vi "G Code Commands.vi"(4 "Previous G Code":T1, 6 "Current G Code":T1, 8 "Error In":errorcluster, 9 "Fast Velocity(mm/s)":dbl=80.0, 10 "Coordinate Space Reference In":refnum<k21>, 11 "Axis Resources In":refnum<k21>[](array[refnum])=["", "", "", ""]) -> (0 "Error Out":errorcluster, 2 "Coordinate Space Reference Out":refnum<k21>, 3 "Axis Resources Out":refnum<k21>[](array[refnum]))   [LabVIEW 2018]
uses:
  Type Defs/G Code Command Cluster.ctl
  Type Defs/The Motion Parameters.ctl
  <vilib>/Motion/Express/_s/nimc.ex.straightLineMove.startStraightLineMove.coordinate.modeAbsolute.blendEnable.1.vi
  <vilib>/Motion/Express/_s/nimc.ex.arcMove.startArcMove.coordinate.modeCircular.blendEnable.1.vi
  <vilib>/Motion/Express/_s/nimc.ex.stopMove.stop.axis.modeDecelerate.vi
  <vilib>/Motion/Express/_s/nimc.ex.resetPosition.resetPosition.axis.vi
  <vilib>/Motion/BlockNode/FB.NIMotion.xnode
  <vilib>/Motion/Express/_s/nimc.fb.straightLineMove.blendMode.ctl
  <vilib>/Motion/Express/_s/nimc.fb.arcMove.blendMode.ctl
panel:
  in  "Dwell Time(ms)":u32
  in  "Motion Parameters":T2={"Timeout"=-1.0, "Blend Mode"=10551335, "Acceleration"=2000.0, "Deceleration"=2000.0, "Accel. Jerk"=20000.0, "Decel. Jerk"=20000.0, "Smoothing"=1.0, "Last Blend"=FALSE, "Blend Delay"=0.0} {"Blend Delay" format="%#_13g"; "Smoothing" format="%#_13g"; "Decel. Jerk" format="%#_13g"; "Accel. Jerk" format="%#_13g"; "Deceleration" format="%#_13g"; "Acceleration" format="%#_13g"; "Blend Mode" items=["At Profile Complete"=10551335, "At Deceleration"=10551334, "After Delay"=10551336]}
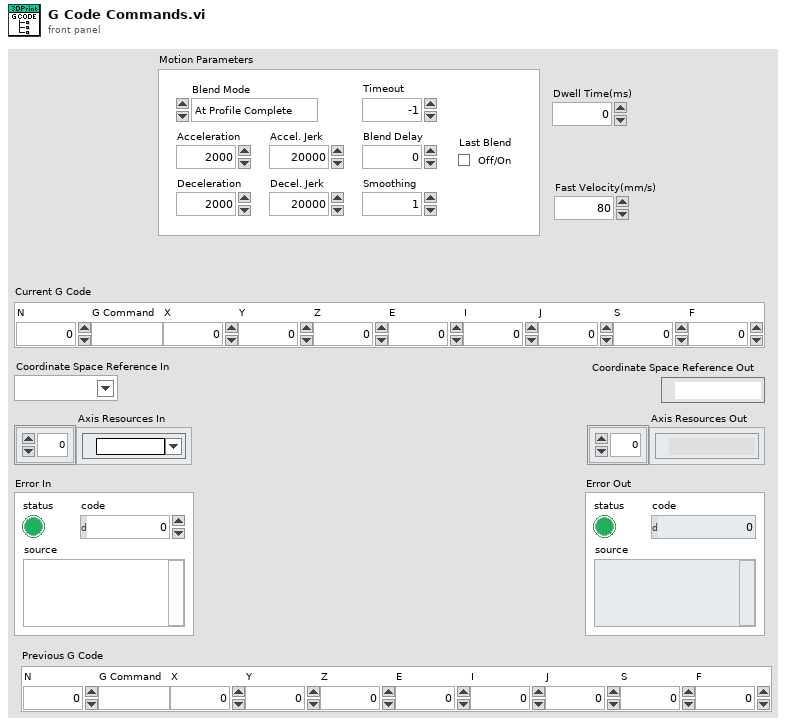
[diagram p1: front panel]
types:
  T1 = typedef "G Code Command Cluster.ctl" = cluster{"N":dbl, "G Command":string, "X":dbl, "Y":dbl, "Z":dbl, "E":dbl, "I":dbl, "J":dbl, "S":dbl, "F":dbl}
  T2 = typedef "The Motion Parameters.ctl" = cluster{"Timeout":dbl, "Blend Mode":i32, "Acceleration":dbl, "Deceleration":dbl, "Accel. Jerk":dbl, "Decel. Jerk":dbl, "Smoothing":dbl, "Last Blend":bool, "Blend Delay":dbl}
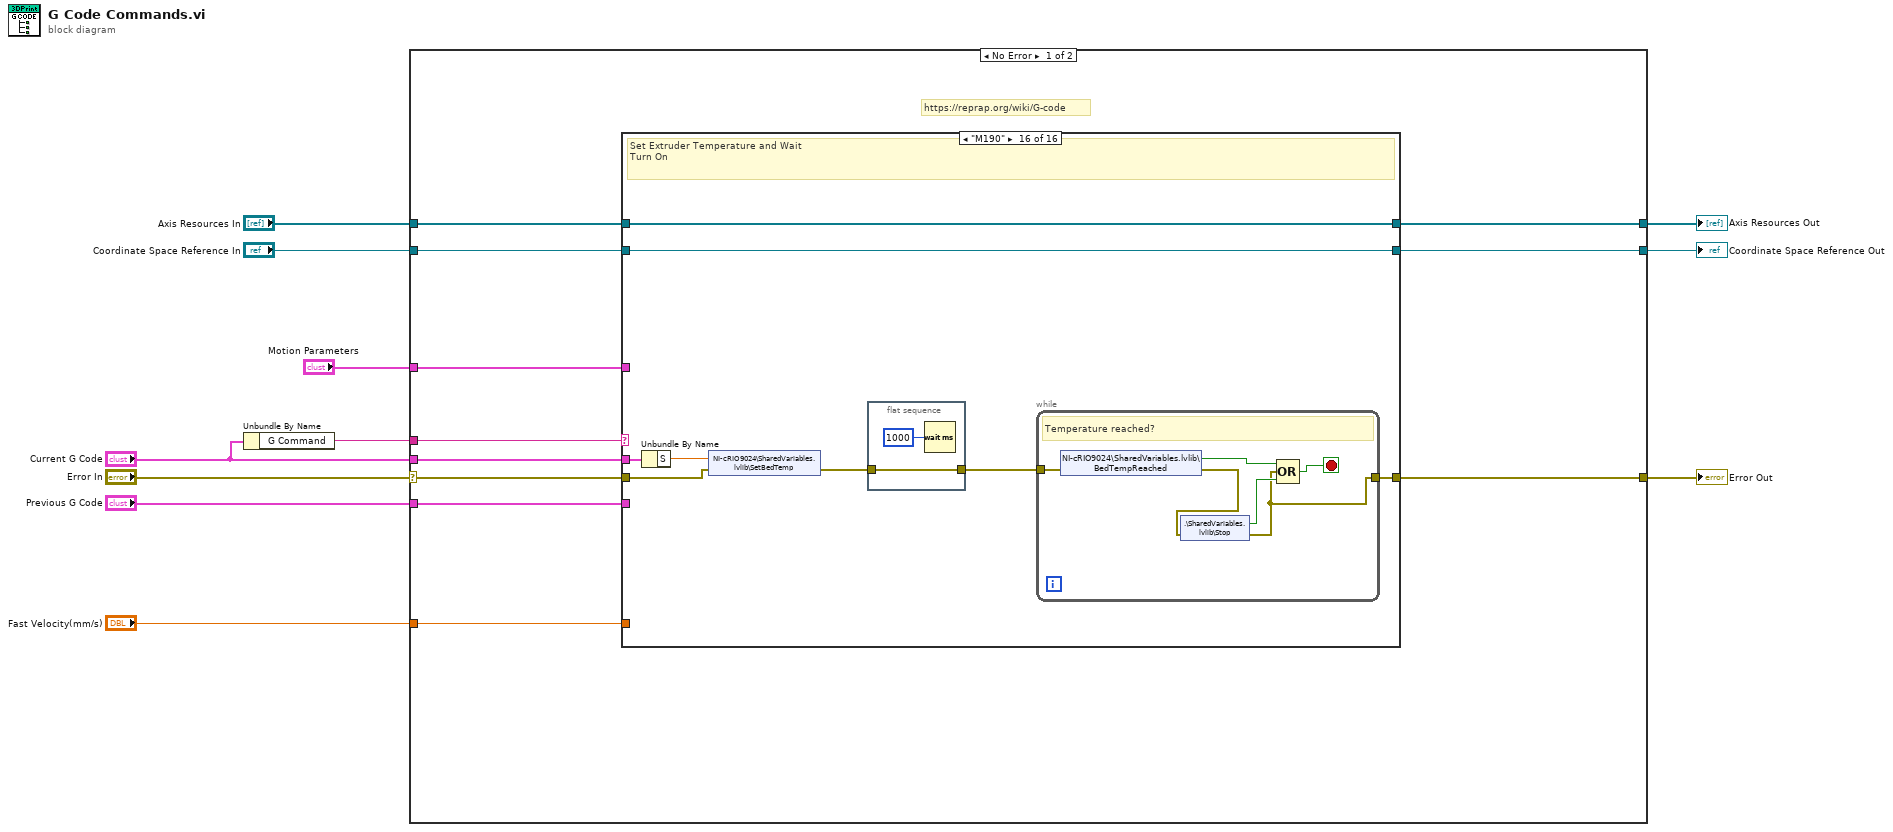
[diagram p0: block diagram]
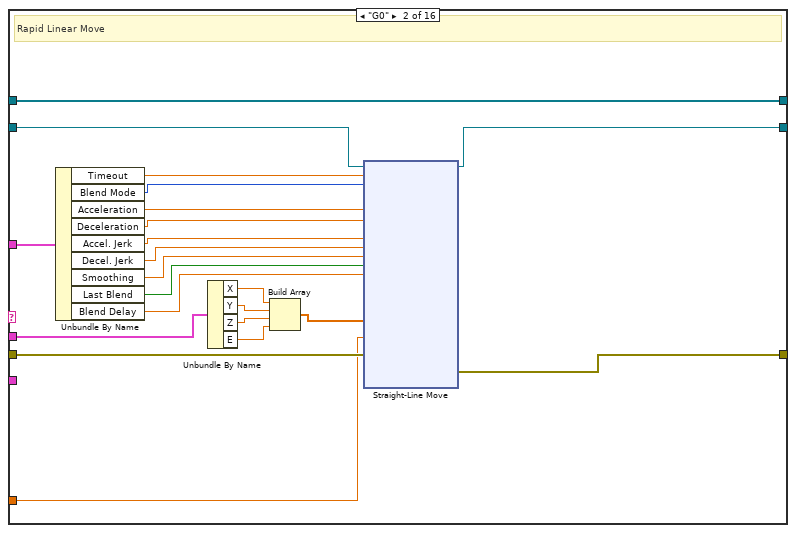
[diagram p3: hidden frame]
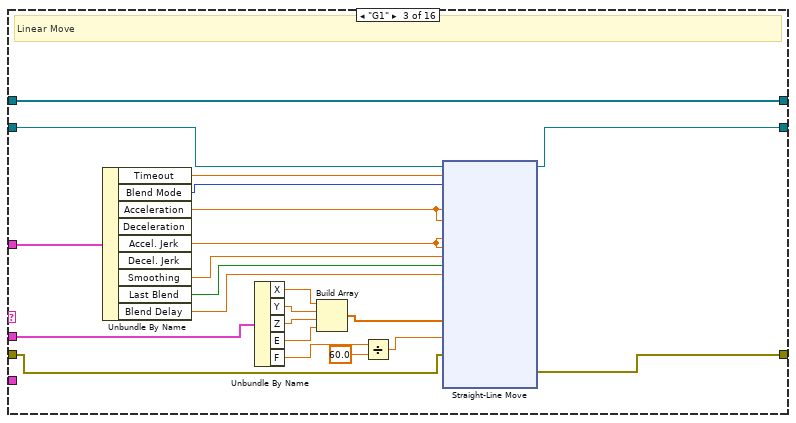
[diagram p4: hidden frame]
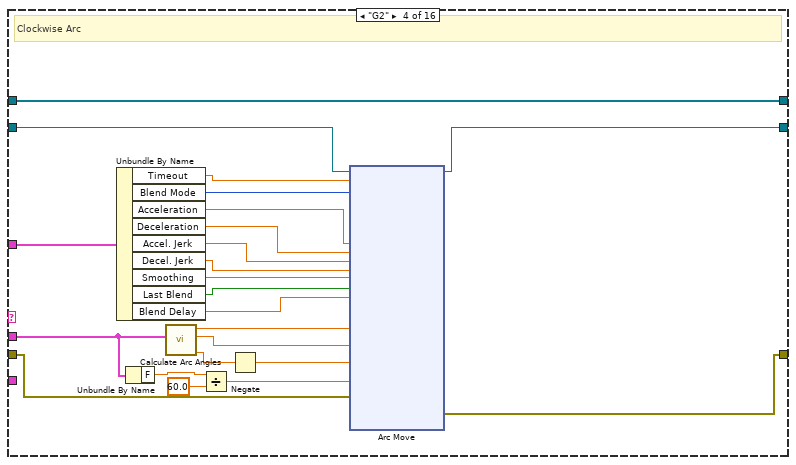
[diagram p5: hidden frame]
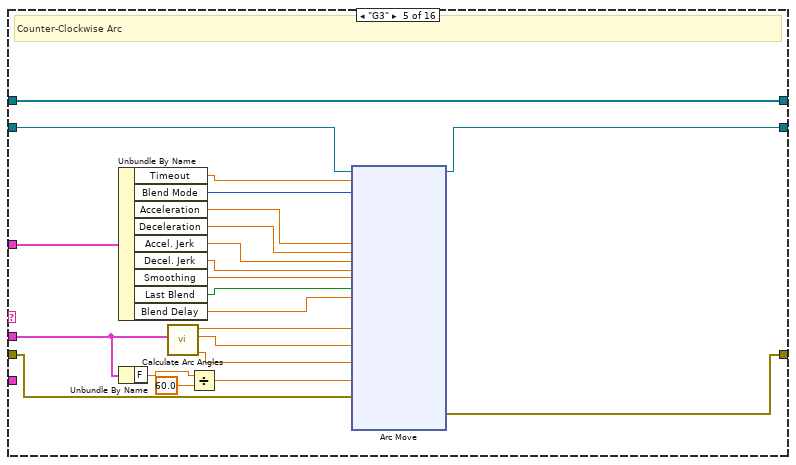
[diagram p6: hidden frame]
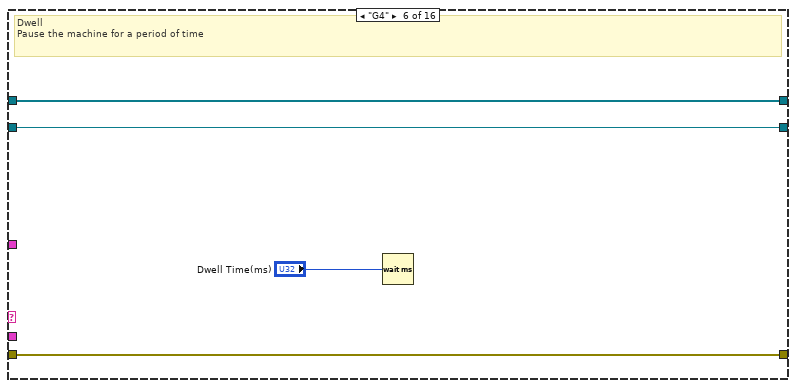
[diagram p7: hidden frame]
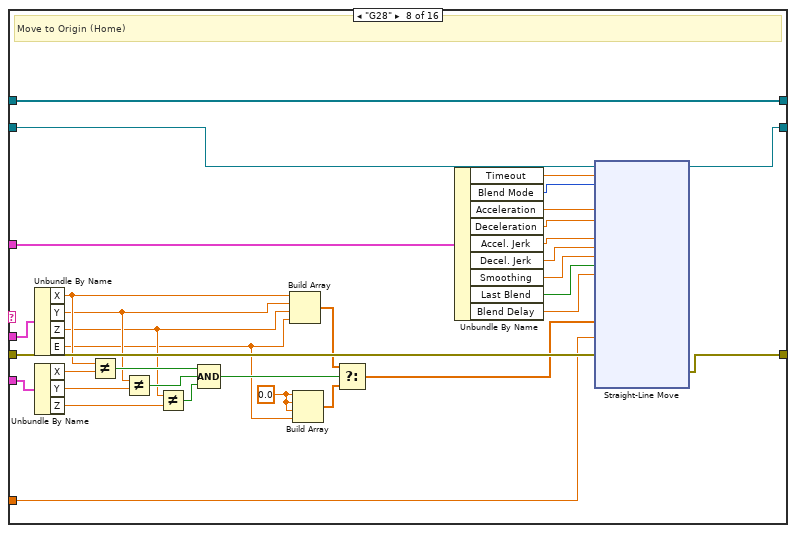
[diagram p9: hidden frame]
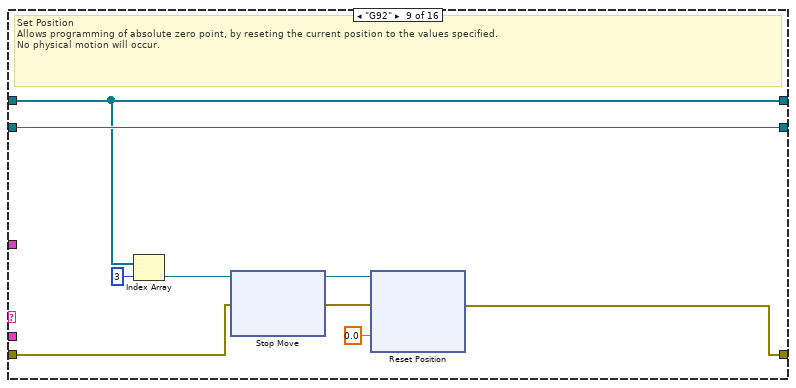
[diagram p10: hidden frame]
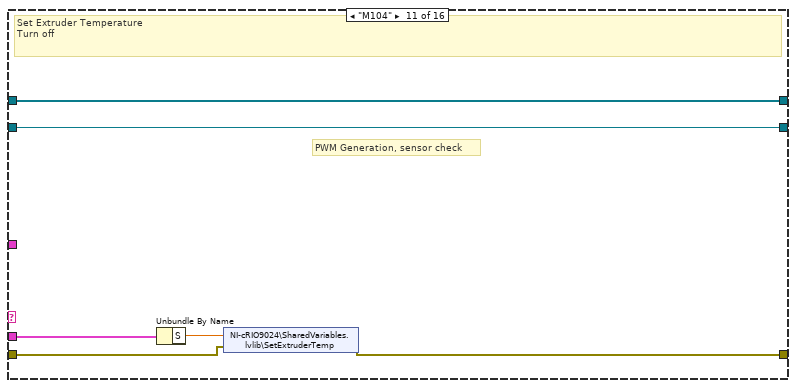
[diagram p12: hidden frame]
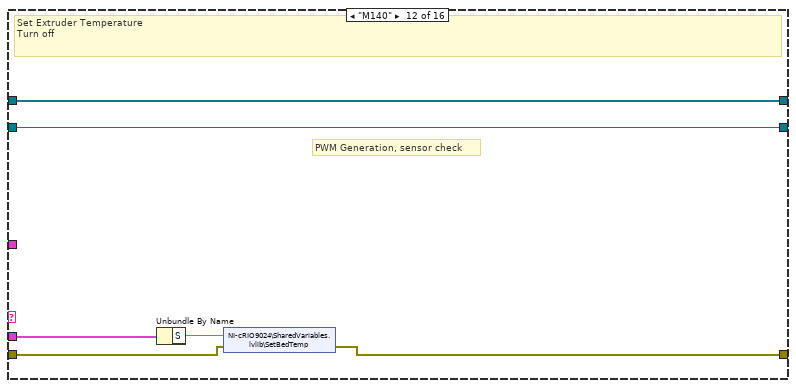
[diagram p13: hidden frame]
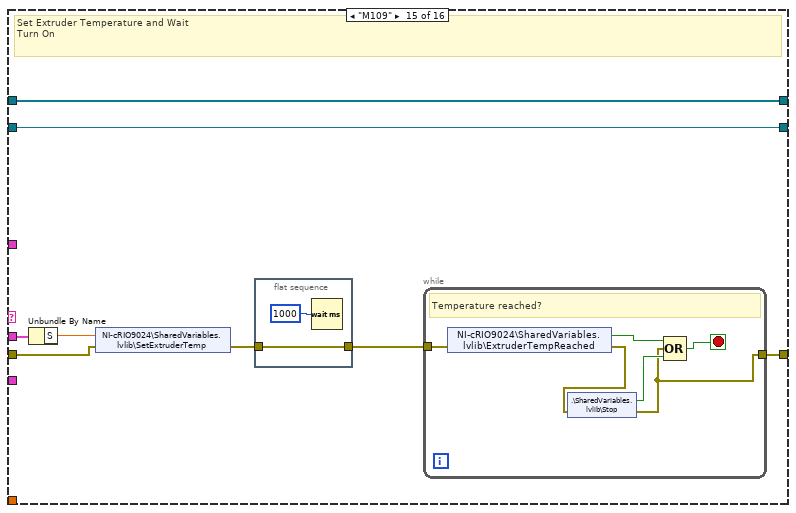
[diagram p16: hidden frame]
diagram:
  n1 = Unbundle By Name("Current G Code") -> ("G Command"=w7:string)
  n2 = case shown="No Error" "Error In" {
    selector: "Error In" -> [w19 w336]
    tunnel: w7 -> [w22 _]
    tunnel: "Axis Resources In" -> [w21 w334]
    tunnel: [w18 w336] -> w9
    tunnel: "Motion Parameters" -> [w20 _]
    tunnel: "Current G Code" -> [w17 _]
    tunnel: "Coordinate Space Reference In" -> [w16 w335]
    tunnel: [w15 w335] -> w4
    tunnel: [w14 w334] -> w3
    tunnel: "Previous G Code" -> [w13 _]
    tunnel: "Fast Velocity(mm/s)" -> [w12 _]
    frame No Error {
      # "https://reprap.org/wiki/G-code"
      n3 = case shown="\"M190\"" w22 {
        tunnel: w21 -> [w23 w26 w73 w113 w158 w199 w203 w232 w264 w281 w284 w290 w296 w299 w304 w320]
        tunnel: w20 -> [_ w47 w80 w132 w164 _ _ w237 _ _ _ _ _ _ _ _]
        tunnel: w19 -> [w25 w37 w77 w115 w162 w202 w205 w236 w259 w283 w287 w293 w298 w301 w307 w323]
        tunnel: [w25 w36 w76 w131 w160 w202 w205 w235 w266 w283 w286 w292 w298 w301 w306 w322] -> w18
        tunnel: w17 -> [_ w35 w79 w116 w161 _ _ w231 _ _ w288 w294 _ _ w309 w325]
        tunnel: w16 -> [w24 w30 w78 w130 w163 w200 w204 w238 w265 w282 w285 w291 w297 w300 w305 w321]
        tunnel: w12 -> [_ w28 _ _ _ _ _ w234 _ _ _ _ _ _ _ _]
        tunnel: [w24 w27 w74 w114 w159 w200 w204 w233 w265 w282 w285 w291 w297 w300 w305 w321] -> w15
        tunnel: [w23 w26 w73 w113 w158 w199 w203 w232 w264 w281 w284 w290 w296 w299 w304 w320] -> w14
        tunnel: w13 -> [_ _ _ _ _ _ _ w230 _ _ _ _ _ _ _ _]
        frame Default {
          # "Place Holder fo other steps"
        }
        frame "G0" {
          # "Rapid Linear Move"
          n4 = Unbundle By Name(w47) -> ("Timeout"=w38:dbl, "Blend Mode"=w39:i32, "Acceleration"=w40:dbl, "Deceleration"=w41:dbl, "Accel. Jerk"=w42:dbl, "Decel. Jerk"=w43:dbl, "Smoothing"=w44:dbl, "Last Blend"=w45:bool, "Blend Delay"=w46:dbl)
          n5 = Unbundle By Name(w35) -> ("X"=w31:dbl, "Y"=w34:dbl, "Z"=w32:dbl, "E"=w33:dbl)
          n6 = Build Array(w31, w34, w32, w33) -> (w29:dbl[])
          n7 = xnode ("Straight-Line Move")("position[]"=w29, "velocity"=w28, "error in"=w37, "resource"=w30, "timeout"=w38, "blend mode"=w39, "acceleration"=w40, "deceleration"=w41, "accel. jerk"=w42, "decel. jerk"=w43, "smoothing"=w44, "last blend"=w45, "blend delay"=w46) -> ("error out"=w36:errorcluster, "resource out"=w27:refnum<k21>)  [unwired: 1 out]
        }
        frame "G1" {
          # "Linear Move"
          n8 = Unbundle By Name(w80) -> ("Timeout"=w85:dbl, "Blend Mode"=w86:i32, "Acceleration"=w69:dbl, "Accel. Jerk"=w68:dbl, "Smoothing"=w87:dbl, "Last Blend"=w88:bool, "Blend Delay"=w89:dbl)  [unwired: 2 out]
          n9 = Unbundle By Name(w79) -> ("X"=w81:dbl, "Y"=w84:dbl, "Z"=w82:dbl, "E"=w83:dbl, "F"=w72:dbl)
          n10 = Build Array(w81, w84, w82, w83) -> (w75:dbl[])
          n11 = Divide(x=w72, y=60.0) -> (x/y=w70:dbl)
          n12 = xnode ("Straight-Line Move")("position[]"=w75, "velocity"=w70, "error in"=w77, "resource"=w78, "timeout"=w85, "blend mode"=w86, "acceleration"=w69, "deceleration"=w69, "accel. jerk"=w68, "decel. jerk"=w68, "smoothing"=w87, "last blend"=w88, "blend delay"=w89) -> ("error out"=w76:errorcluster, "resource out"=w74:refnum<k21>)  [unwired: 1 out]
        }
        frame "G2" {
          # "Clockwise Arc"
          n13 = Unbundle By Name(w132) -> ("Timeout"=w129:dbl, "Blend Mode"=w128:i32, "Acceleration"=w127:dbl, "Deceleration"=w126:dbl, "Accel. Jerk"=w125:dbl, "Decel. Jerk"=w124:dbl, "Smoothing"=w123:dbl, "Last Blend"=w122:bool, "Blend Delay"=w121:dbl)
          n14 = Unbundle By Name(w116) -> ("F"=w111:dbl)
          n15 = call "Calculate Arc Angles.vi"("Arc CMD"=w116) -> ("travel angle out"=w120:dbl, "start angle (tangent)"=w118:dbl, "R"=w117:dbl)  [unwired: 8 in]
          n16 = Divide(x=w111, y=60.0) -> (x/y=w110:dbl)
          n17 = Negate(x=w120) -> (-x=w119:dbl)
          n18 = xnode ("Arc Move")("radius"=w117, "start angle"=w118, "travel angle"=w119, "velocity"=w110, "error in"=w115, "resource"=w130, "timeout"=w129, "blend mode"=w128, "acceleration"=w127, "deceleration"=w126, "accel. jerk"=w125, "decel. jerk"=w124, "smoothing"=w123, "last blend"=w122, "blend delay"=w121) -> ("error out"=w131:errorcluster, "resource out"=w114:refnum<k21>)  [unwired: 1 out]
        }
        frame "G3" {
          # "Counter-Clockwise Arc"
          n19 = Unbundle By Name(w164) -> ("Timeout"=w176:dbl, "Blend Mode"=w175:i32, "Acceleration"=w174:dbl, "Deceleration"=w173:dbl, "Accel. Jerk"=w172:dbl, "Decel. Jerk"=w171:dbl, "Smoothing"=w170:dbl, "Last Blend"=w169:bool, "Blend Delay"=w168:dbl)
          n20 = Unbundle By Name(w161) -> ("F"=w156:dbl)
          n21 = call "Calculate Arc Angles.vi"("Arc CMD"=w161) -> ("travel angle out"=w167:dbl, "start angle (tangent)"=w166:dbl, "R"=w165:dbl)  [unwired: 8 in]
          n22 = Divide(x=w156, y=60.0) -> (x/y=w155:dbl)
          n23 = xnode ("Arc Move")("radius"=w165, "start angle"=w166, "travel angle"=w167, "velocity"=w155, "error in"=w162, "resource"=w163, "timeout"=w176, "blend mode"=w175, "acceleration"=w174, "deceleration"=w173, "accel. jerk"=w172, "decel. jerk"=w171, "smoothing"=w170, "last blend"=w169, "blend delay"=w168) -> ("error out"=w160:errorcluster, "resource out"=w159:refnum<k21>)  [unwired: 1 out]
        }
        frame "G4" {
          # "Dwell\nPause the machine for a period of time"
          n24 = Wait (ms)(milliseconds to wait="Dwell Time(ms)") -> ()  [unwired: 1 out]
        }
        frame "G21" {
          # "Set Units to Millimeters"
        }
        frame "G28" {
          w207 = 0.0 ("element")
          # "Move to Origin (Home)"
          n25 = Unbundle By Name(w231) -> ("X"=w214:dbl, "Y"=w213:dbl, "Z"=w212:dbl, "E"=w208:dbl)
          n26 = Unbundle By Name(w230) -> ("X"=w229:dbl, "Y"=w228:dbl, "Z"=w227:dbl)
          n27 = Not Equal?(x=w214, y=w229) -> (x != y?=w224:bool)
          n28 = Not Equal?(x=w213, y=w228) -> (x != y?=w225:bool)
          n29 = Not Equal?(x=w212, y=w227) -> (x != y?=w226:bool)
          n30 = Compound Arithmetic op=AND(w224, w225, w226) -> (w211:bool)
          n31 = Build Array(w214, w213, w212, w208) -> (w210:dbl[])
          n32 = Build Array(w207, w207, w207, w208) -> (w209:dbl[])
          n33 = Select(t=w210, s=w211, f=w209) -> (s? t:f=w206:dbl[])
          n34 = Unbundle By Name(w237) -> ("Timeout"=w215:dbl, "Blend Mode"=w216:i32, "Acceleration"=w217:dbl, "Deceleration"=w218:dbl, "Accel. Jerk"=w219:dbl, "Decel. Jerk"=w220:dbl, "Smoothing"=w221:dbl, "Last Blend"=w222:bool, "Blend Delay"=w223:dbl)
          n35 = xnode ("Straight-Line Move")("position[]"=w206, "velocity"=w234, "error in"=w236, "resource"=w238, "timeout"=w215, "blend mode"=w216, "acceleration"=w217, "deceleration"=w218, "accel. jerk"=w219, "decel. jerk"=w220, "smoothing"=w221, "last blend"=w222, "blend delay"=w223) -> ("error out"=w235:errorcluster, "resource out"=w233:refnum<k21>)  [unwired: 1 out]
        }
        frame "G92" {
          # "Set Position\nAllows programming of absolute zero point, by reseting the current position to the values specified. \nNo physical motion will occur."
          n36 = Index Array(array=w264, index=3) -> (element=w263:refnum<k21>)
          n37 = xnode ("Stop Move")("resource"=w263, "error in"=w259) -> ("resource out"=w262:refnum<k21>, "error out"=w260:errorcluster)  [unwired: 1 in, 1 out]
          n38 = xnode ("Reset Position")("position"=0.0, "resource"=w262, "error in"=w260) -> ("error out"=w266:errorcluster)  [unwired: 1 out]
        }
        frame "M82" {
          # "Set extruder to absolute mode\nSets the extruder (E-axis) to absolute or relative positioning"
        }
        frame "M104" {
          # "PWM Generation, sensor check"
          # "Set Extruder Temperature\nTurn off"
          n39 = Unbundle By Name(w288) -> ("S"=w289:dbl)
          n40 = shared-variable "NI-cRIO9024\\SharedVariables.lvlib\\SetExtruderTemp"(w289, error in=w287) -> (error out=w286:errorcluster)
        }
        frame "M140" {
          # "PWM Generation, sensor check"
          # "Set Extruder Temperature\nTurn off"
          n41 = Unbundle By Name(w294) -> ("S"=w295:dbl)
          n42 = shared-variable "NI-cRIO9024\\SharedVariables.lvlib\\SetBedTemp"(w295, error in=w293) -> (error out=w292:errorcluster)
        }
        frame "M106" {
          # "Fan On\n Turns on the cooling fan."
        }
        frame "M107" {
          # "Fan Off\n Turns off the cooling fan."
        }
        frame "M109" {
          # "Set Extruder Temperature and Wait\nTurn On"
          n43 = Unbundle By Name(w309) -> ("S"=w308:dbl)
          n44 = shared-variable "NI-cRIO9024\\SharedVariables.lvlib\\SetExtruderTemp"(w308, error in=w307) -> (error out=w303:errorcluster)
          n45 = flat-sequence {
            tunnel: w303 -> [w310]
            tunnel: [w310] -> w302
            frame #0 {
              n46 = Wait (ms)(milliseconds to wait=u32 1000) -> ()  [unwired: 1 out]
            }
          }
          n47 = while {
            tunnel: w302 -> [w317]
            tunnel: [w312] -> w306
            stop <- w316 stop-if-true
            # "Temperature reached?"
            n48 = shared-variable "NI-cRIO9024\\SharedVariables.lvlib\\ExtruderTempReached"(error in=w317) -> (w315:bool, error out=w313:errorcluster)
            n49 = shared-variable ".\\SharedVariables.lvlib\\Stop"(error in=w313) -> (w314:bool, error out=w312:errorcluster)
            n50 = Compound Arithmetic op=OR(w315, w312, w314) -> (w316:bool)
          }
        }
        frame "M190" {
          # "Set Extruder Temperature and Wait\nTurn On"
          n51 = Unbundle By Name(w325) -> ("S"=w324:dbl)
          n52 = shared-variable "NI-cRIO9024\\SharedVariables.lvlib\\SetBedTemp"(w324, error in=w323) -> (error out=w319:errorcluster)
          n53 = flat-sequence {
            tunnel: w319 -> [w326]
            tunnel: [w326] -> w318
            frame #0 {
              n54 = Wait (ms)(milliseconds to wait=u32 1000) -> ()  [unwired: 1 out]
            }
          }
          n55 = while {
            tunnel: w318 -> [w333]
            tunnel: [w328] -> w322
            stop <- w332 stop-if-true
            # "Temperature reached?"
            n56 = shared-variable "NI-cRIO9024\\SharedVariables.lvlib\\BedTempReached"(error in=w333) -> (w331:bool, error out=w329:errorcluster)
            n57 = shared-variable ".\\SharedVariables.lvlib\\Stop"(error in=w329) -> (w330:bool, error out=w328:errorcluster)
            n58 = Compound Arithmetic op=OR(w331, w328, w330) -> (w332:bool)
          }
        }
      }
    }
    frame Error {
    }
  }
  "Error Out" <- w9
  "Coordinate Space Reference Out" <- w4
  "Axis Resources Out" <- w3
